vi "SpeedArrays.vi"(11 "Motor Speeds":T1={"M1 Speed"=1.0, "M4 Speed"=0.0}) -> (3 "Motor Speeds":dbl[](array[numeric]))   [LabVIEW 2014]
uses:
  controls/MotorSpeeds.ctl
panel:
  # "This one only works for doubles"
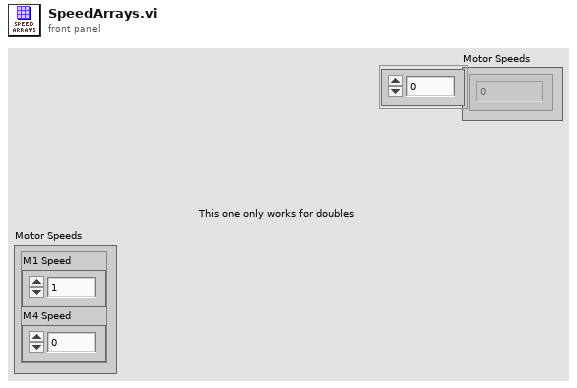
[diagram p1: front panel]
types:
  T1 = typedef "MotorSpeeds.ctl" = cluster{"M1 Speed":dbl, "M4 Speed":dbl}
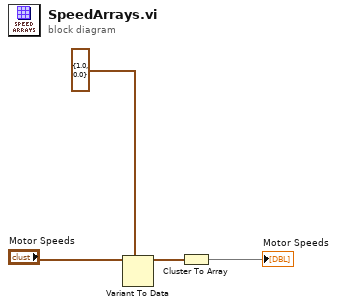
[diagram p0: block diagram]
diagram:
  n1 = Variant To Data(type=T1 {"M1 Speed"=1.0, "M4 Speed"=0.0} ("Motor Speeds"), Variant="Motor Speeds") -> (data=w4:T1)  [unwired: 1 in, 1 out]
  n2 = Cluster To Array(cluster=w4) -> (array=→"Motor Speeds":dbl[])
